vi "p13.vi"() -> ()   [LabVIEW 2015]
panel:
  out "Ring":u16(ring) items=["12s", "45h", "7r"]
  out "Logical Shift (-2)":u16 format="%016b"
  out "floor(x)":dbl
  out "abs(x)":dbl
  out "ceil(x)":dbl
  out "Machine Epsilon":dbl=2.220446049250313e-16
  out "-Inf":dbl=-inf
  out "overflow?":bool
  out "FXP with overflow removed":fxp<+,1,0>
  out "FXP with overflow included":fxp<+/-,32,16>
  out "overflow?":bool
  out "FXP with overflow cleared":fxp<+,1,0>
  out "r * e^(i*theta)":cdb
  out "x - iy":cdb
  out "Rotate left (-2)":u16 format="%016b"
  out "exponent":dbl
  out "mantissa":dbl
  out "-1, 0, 1":dbl
  out "string":string
  out "String --> Byte array":u8[](array[numeric])
  out "RGB --> Color":u32(colorbox)
  out "B":u8
  out "G":u8
  out "R":u8
  out "Resolved Color":u32 format="%.0x"
  in  "Color Box":u32(colorbox)
  out "Change Unit Base":dbl[unit]
  out "Convert Unit":dbl[unit]
  out "Time Stamp":timestamp
  # "TO TIMESTAMP"
  # "POLAR TO COMPLEX"
  # "CONSTANTS"
  # "SIGN"
  # "CONVERT UNIT"
  # "MANTISSA & EXPONENT"
  # "CEIL , ABS , FLOOR"
  # "CAST UNIT BASES"
  # "COLOR TO RGB"
  # "ROTATE"
  # "LOGICAL SHIFT"
  # "RING CONSTANT"
  # "COMPLEX CONJUGATE"
  # "RGB TO COLOR"
  # "FXP & CLEAR OVERFLOW"
  # "STRING TO BYTE ARRAY"
  # "FXP - OVERFLOW INCLUDED"
  # "FXP - OVERFLOW REMOVED"
  # "BYTE ARRAY TO STRING"
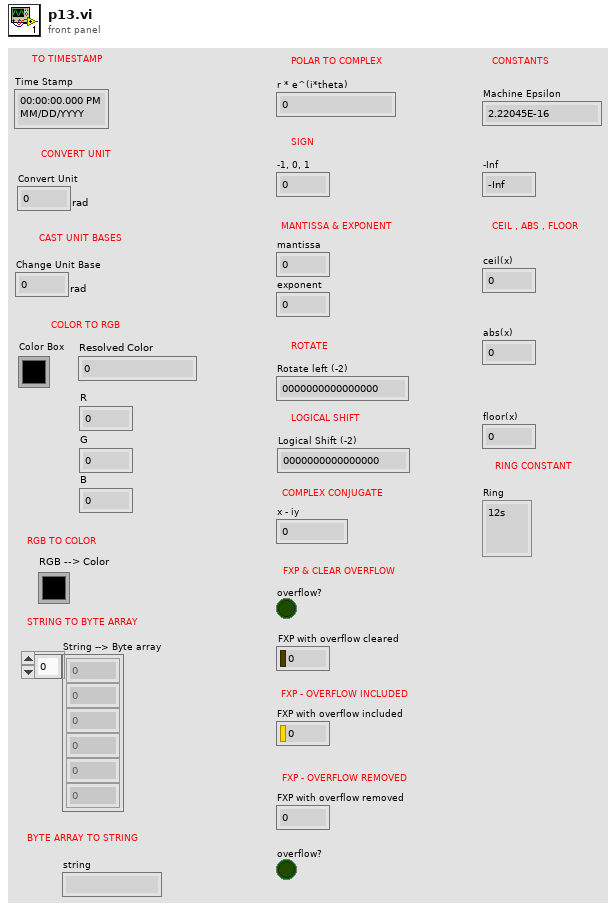
[diagram p1: front panel]
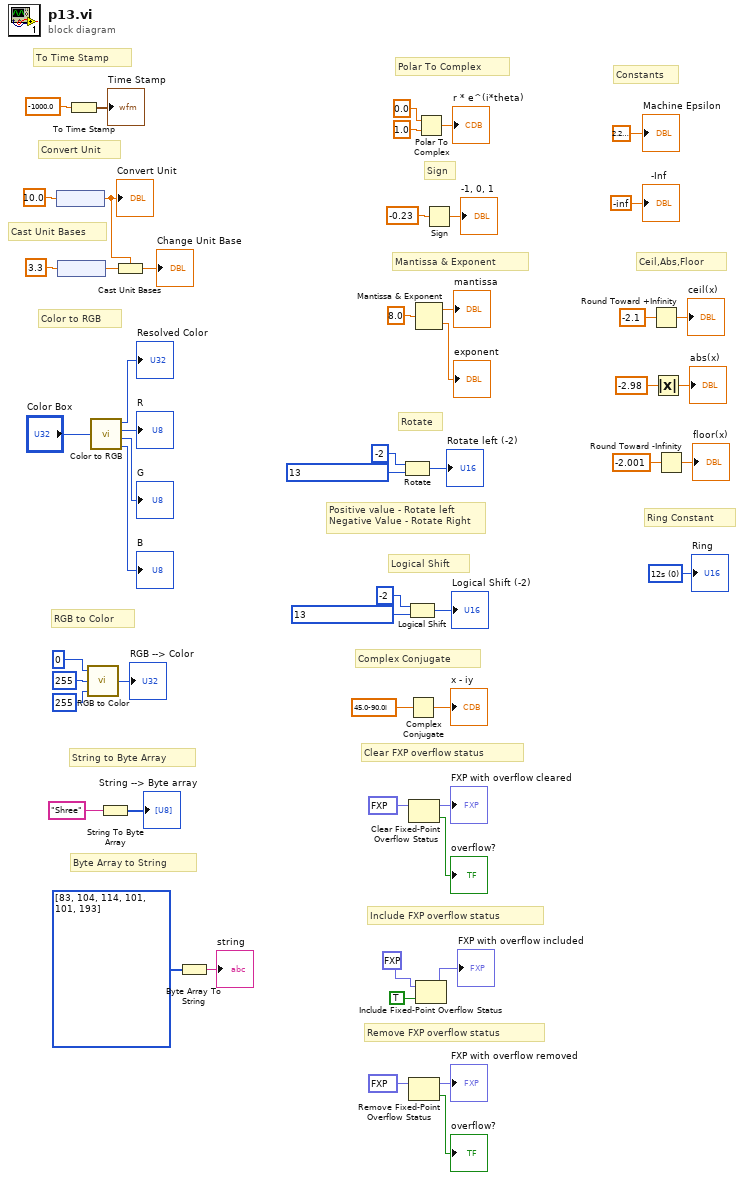
[diagram p0: block diagram]
diagram:
  w1 = u16 0 items=["12s", "45h", "7r"]
  # "Ring Constant"
  # "Ceil,Abs,Floor"
  # "Constants"
  # "Remove FXP overflow status"
  # "Include FXP overflow status"
  # "Clear FXP overflow status"
  # "Complex Conjugate"
  # "Logical Shift"
  # "Rotate"
  # "Byte Array to String"
  # "String to Byte Array"
  # "Mantissa & Exponent"
  # "Sign"
  # "Polar To Complex"
  # "RGB to Color"
  # "Color to RGB"
  # "Cast Unit Bases"
  # "Convert Unit"
  # "To Time Stamp"
  # "Positive value - Rotate left\nNegative Value - Rotate Right"
  n1 = node(10.0) -> (w50:dbl[unit])
  "Convert Unit" <- w50
  n2 = node(3.3 ("x")) -> (w48:dbl[unit])
  n3 = To Time Stamp(1:-1000.0 ("number")) -> (0:→"Time Stamp":timestamp)
  n4 = call <vilib>:"RGB to Color.vi"("B"=u8 255 ("R"), "G"=u8 255 ("R"), "R"=u8 0) -> ("Color"=→"RGB --> Color":u32)
  n5 = call <vilib>:"Color to RGB.vi"("Color"="Color Box") -> ("Resolved Color"=→"Resolved Color":u32, "R"=→"R":u8, "G"=→"G":u8, "B"=→"B":u8)
  n6 = String To Byte Array(string="Shree") -> (unsigned byte array=→"String --> Byte array":u8[])
  n7 = Cast Unit Bases(0:w48, 1:w50) -> (2:→"Change Unit Base":dbl[unit])
  n8 = Byte Array To String(unsigned byte array=u8[] [83, 104, 114, 101, 101, 193] ("unsigned byte array 2")) -> (string=→"string":string)
  n9 = Rotate(1:u16 13 ("x"), 2:i16 -2 ("y")) -> (0:→"Rotate left (-2)":u16)
  n10 = Logical Shift(y=i16 -2, x=u16 13) -> (x << y=→"Logical Shift (-2)":u16)
  n11 = Complex Conjugate(1:cdb 45.0-90.0i ("x + iy")) -> (0:→"x - iy":cdb)
  n12 = Clear Fixed-Point Overflow Status(3:fxp<+,1,0> data[9B] ("FXP")) -> (0:→"overflow?":bool, 1:→"FXP with overflow cleared":fxp<+,1,0>)
  n13 = Remove Fixed-Point Overflow Status(3:fxp<+,1,0> data[9B] ("FXP")) -> (0:→"overflow?":bool, 1:→"FXP with overflow removed":fxp<+,1,0>)
  n14 = Mantissa & Exponent(0:8.0 ("number")) -> (1:→"mantissa":dbl, 2:→"exponent":dbl)
  n15 = Polar To Complex(1:1.0 ("theta"), 2:0.0 ("r")) -> (0:→"r * e^(i*theta)":cdb)
  n16 = Include Fixed-Point Overflow Status(2:TRUE ("overflow"), 3:fxp<+/-,32,16> 0.0 ("FXP")) -> (1:→"FXP with overflow included":fxp<+/-,32,16>)
  n17 = Sign(1:-0.23 ("number")) -> (0:→"-1, 0, 1":dbl)
  n18 = Round Toward +Infinity(x=-2.1) -> (ceil(x): smallest int >= x=→"ceil(x)":dbl)
  n19 = Absolute Value(x=-2.98) -> (abs(x)=→"abs(x)":dbl)
  n20 = Round Toward -Infinity(1:-2.001 ("x")) -> (0:→"floor(x)":dbl)
  "-Inf" <- -inf
  "Machine Epsilon" <- 2.220446049250313e-16
  "Ring" <- w1
